vi "DHE_GetActiveDevice.vi"() -> (7 "DHE_ActiveDevice":string)   [LabVIEW 2016]
uses:
  private/vis/DHE_GBLDriverVariables.vi
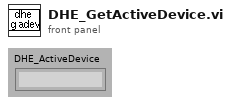
[diagram p1: front panel]
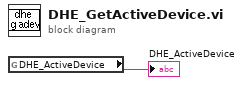
[diagram p0: block diagram]
diagram:
  n1 = global read "DHE_GBLDriverVariables.vi" "DHE_ActiveDevice"() -> (→"DHE_ActiveDevice":string)
